vi "get project.vi"(8 "error in (no error)":errorcluster, 11 "path":string) -> (0 "error out":errorcluster, 3 "text":string)   [LabVIEW 2020]
doc: "Returns the XML content of a LabVIEW Project- or Library-File specified by path. (lvlib, lvproj, lvclass filetypes). To get a full projects multiple calls may be necessary to get all nested libraries."
uses:
  G-AI Core/G-AI Core.lvlib
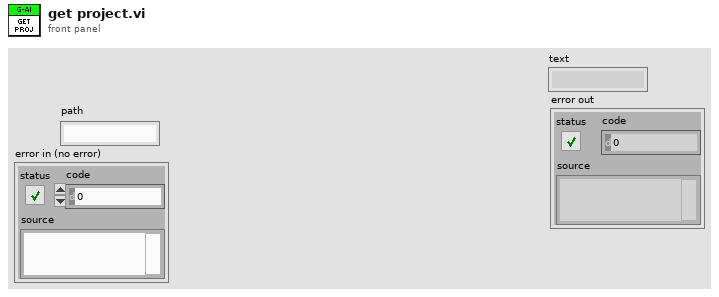
[diagram p1: front panel]
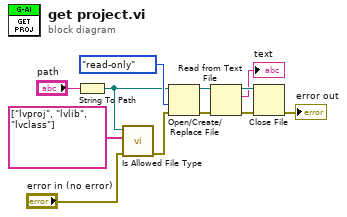
[diagram p0: block diagram]
diagram:
  n1 = String To Path(string="path") -> (path=w4:path)
  n2 = call "Is Allowed File Type.vi"("error in (no error)"="error in (no error)", "y"=string[] ["lvproj", "lvlib", "lvclass"], "Path"=w4) -> ("error out"=w3:errorcluster)  [unwired: 8 in]
  n3 = Open/Create/Replace File(file path (use dialog)=w4, error in=w3, access (0:read/write)=enum16{"read/write", "read-only", "write-only"}."read-only") -> (refnum out=w11:refnum<file>, error out=w10:errorcluster)  [unwired: 3 in, 1 out]
  n4 = Read from Text File(file (use dialog)=w11, error in=w10) -> (refnum out=w9:refnum<file>, text=→"text":string, error out=w8:errorcluster)  [unwired: 2 in, 1 out]
  n5 = Close File(refnum=w9, error in=w8) -> (error out=→"error out":errorcluster)  [unwired: 1 out]
